vi "ep_Read Samples Count.vi"(8 "error in (no error)":errorcluster, 11 "system info in":refnum<class "EP System Info.lvclass">) -> (0 "error out":errorcluster, 1 "half-cycle (samples)":i32, 2 "basic calc. interval (samples)":i32, 3 "system info out":refnum<class "EP System Info.lvclass">, 4 "cycles per interval":i32)   [LabVIEW 2011, in "NI_EP_Power Quality.lvlib" / "EP System Info.lvclass"]
uses:
  <vilib>/addons/Electrical Power/PQ/Common/Classes/System Info/EP System Info.lvclass
  <vilib>/addons/Electrical Power/PQ/Common/Classes/System Info/EP System Info.lvclass/EP System Info.ctl
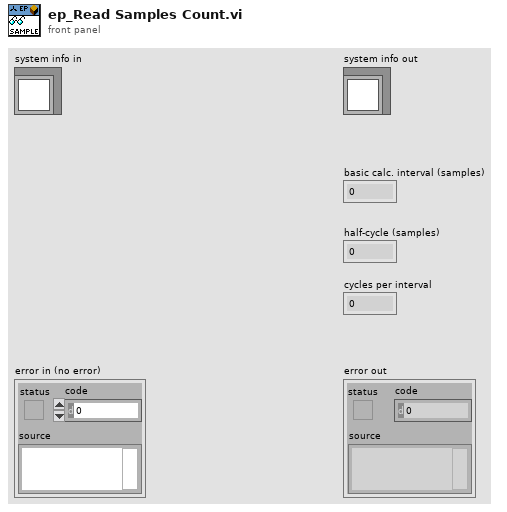
[diagram p1: front panel]
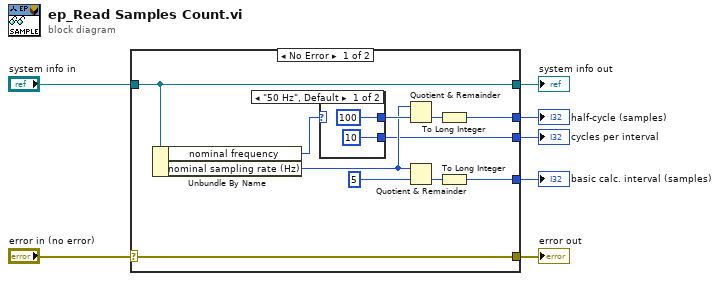
[diagram p0: block diagram]
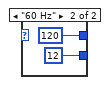
[diagram p2: hidden frame]
diagram:
  n1 = case shown="No Error" "error in (no error)" {
    selector: "error in (no error)" -> [w18 w23]
    tunnel: [w18 w23] -> w6
    tunnel: [w17 w24] -> w4
    tunnel: "system info in" -> [w17 w24]
    tunnel: [w14 _] -> w3
    tunnel: [w10 _] -> w2
    tunnel: [w8 _] -> w1
    frame No Error {
      n2 = Unbundle By Name(w17) -> ("nominal frequency"=w13:enum16{"50 Hz", "60 Hz"}, "nominal sampling rate (Hz)"=w9:u16)
      n3 = case shown="\"50 Hz\", Default" w13 {
        tunnel: [u16 100 ("y") u16 120 ("y")] -> w12
        tunnel: [10 ("y") 12 ("y")] -> w8
        frame "50 Hz", Default {
        }
        frame "60 Hz" {
        }
      }
      n4 = Quotient & Remainder(x=w9, y=w12) -> (floor(x/y)=w11:u16)  [unwired: 1 out]
      n5 = Quotient & Remainder(x=w9, y=u16 5) -> (floor(x/y)=w15:u16)  [unwired: 1 out]
      n6 = To Long Integer(number=w11) -> (32bit integer=w10:i32)
      n7 = To Long Integer(number=w15) -> (32bit integer=w14:i32)
    }
    frame Error {
    }
  }
  "error out" <- w6
  "system info out" <- w4
  "basic calc. interval (samples)" <- w3
  "half-cycle (samples)" <- w2
  "cycles per interval" <- w1
